vi "Current Date & Time String.vi"(8 "Error In":errorcluster, 9 "want seconds? (T)":bool=TRUE, 11 "date format (0)":enum16{"short", "long", "abbreviated"}(ring)) -> (0 "Error Out":errorcluster, 2 "time string":string, 3 "date string":string)   [LabVIEW 2021, in "Strings.lvlib"]
uses:
  Strings/Strings.lvlib
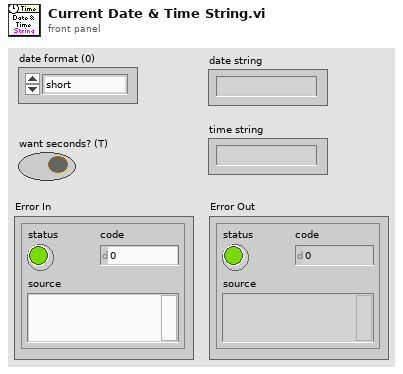
[diagram p1: front panel]
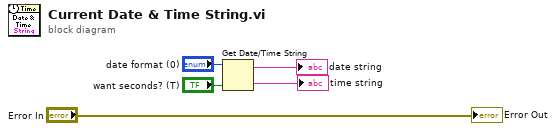
[diagram p0: block diagram]
diagram:
  n1 = Get Date/Time String(date format (0)="date format (0)", want seconds? (F)="want seconds? (T)") -> (date string=→"date string":string, time string=→"time string":string)  [unwired: 1 in]
  "Error Out" <- "Error In"
